vi "Handle Last Ack Core.vi"(4 "error in (no error)":errorcluster, 6 "Last Ack":refnum<class "Last Ack.lvclass">, 7 "CS++BaseActor in":refnum<class "CS++BaseActor.lvclass">) -> (0 "error out":errorcluster, 3 "CS++BaseActor out":refnum<class "CS++BaseActor.lvclass">)   [LabVIEW 2016, in "CS++BaseActor.lvlib" / "CS++BaseActor.lvclass"]
doc: "(<B>Filename</B>: Actor Framework.lvlib:Actor.lvclass:Handle Last Ack Core.vi)\n\nDefines how the caller actor responds to the Last Ack message from a nested actor. The Last Ack message is the final message a nested actor sends to its caller before it shuts down. The message contains information about the final state of the nested actor.\n\nBy default, this method does nothing except return any error the nested actor sent. A descendant class may override this method to define behavior."
uses:
  CS++BaseActor.lvclass
  <vilib>/ActorFramework/LastAck/Last Ack.lvclass
  CS++BaseActor.lvclass/CS++BaseActor.ctl
  <vilib>/ActorFramework/Message Enqueuer/Message Enqueuer.lvclass
  <vilib>/ActorFramework/Actor/Actor.lvclass
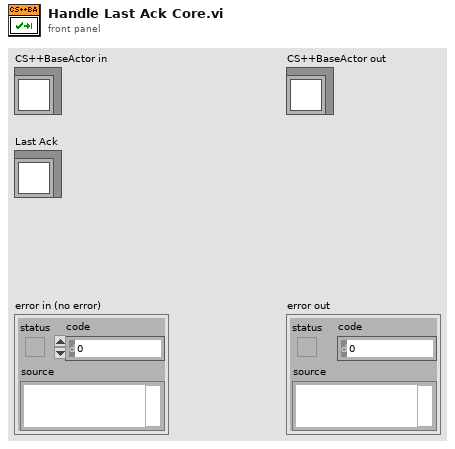
[diagram p1: front panel]
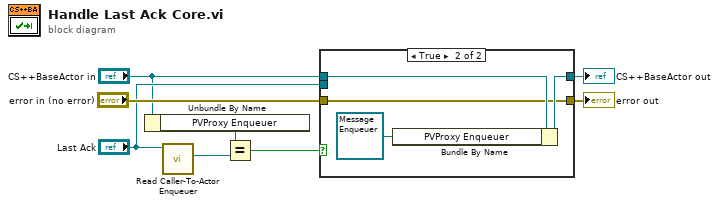
[diagram p0: block diagram]
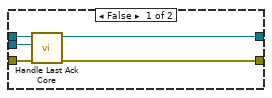
[diagram p2: hidden frame]
diagram:
  n1 = Unbundle By Name("CS++BaseActor in") -> ("PVProxy Enqueuer"=w3:refnum<class "Message Enqueuer.lvclass">)
  n2 = call <vilib>:"Read Caller-To-Actor Enqueuer.vi"("Last Ack"="Last Ack") -> ("Caller-to-Actor Enqueuer"=w2:refnum<class "Message Enqueuer.lvclass">)  [unwired: 10 in]
  n3 = Equal?(x=w3, y=w2) -> (x = y?=w1:bool)
  n4 = case shown="True" w1 {
    tunnel: [w13 w15] -> w8
    tunnel: [w12 w16] -> w7
    tunnel: "error in (no error)" -> [w11 w15]
    tunnel: "Last Ack" -> [w10 _]
    tunnel: "CS++BaseActor in" -> [w9 w17]
    frame False {
      n5 = call-parent "Handle Last Ack Core.vi"("error in (no error)"=w11, "Last Ack"=w10, "Actor in"=w9) -> ("error out"=w13:errorcluster, "Actor out"=w12:refnum<class "CS++BaseActor.lvclass">)  [unwired: 3 in]
    }
    frame True {
      n6 = Bundle By Name(cluster=w17, "PVProxy Enqueuer"=refnum<class "Message Enqueuer.lvclass"> refnum ("PVProxy.PVProxy Enqueuer")) -> (w16:refnum<class "CS++BaseActor.lvclass">)
    }
  }
  "CS++BaseActor out" <- w7
  "error out" <- w8
